vi "create table discretes.vi"(10 "DI table":string[](array[string]), 11 "table name":string="XB") -> (3 "create table parameters":string)   [LabVIEW 2019, in "PostgreSQL.lvlib"]
uses:
  PostgreSQL.lvlib
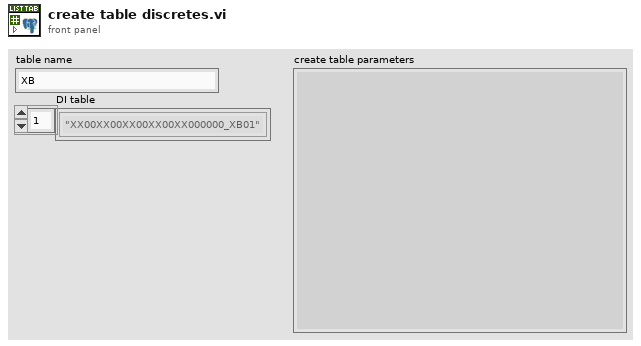
[diagram p1: front panel]
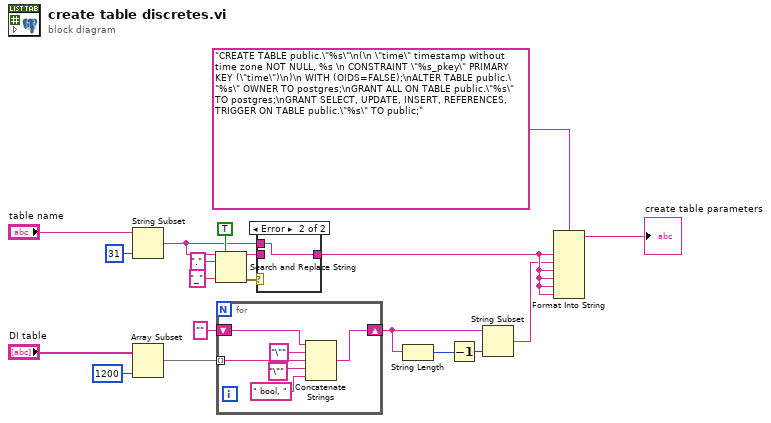
[diagram p0: block diagram]
diagram:
  n1 = String Subset(string="table name", length (rest)=31 ("offset (0)")) -> (substring=w14:string)  [unwired: 1 in]
  n2 = Array Subset(array="DI table", length=1200) -> (w2:string[])  [unwired: 1 in]
  n3 = Search and Replace String(replace all?=TRUE ("replace all? (F)"), input string=w14, search string=".", replace string="_" ("replace string (\"\")")) -> (result string=w16:string, error out=w17:errorcluster)  [unwired: 4 in, 2 out]
  n4 = for {
    tunnel: w2 -> [w23] mode=indexing
    shift-right: [w20] -> w4
    shift-left: "" ("result string") -> [w21]
    n5 = Concatenate Strings(w21, "\"" ("string"), w23, "\"" ("string"), " bool, ") -> (w20:string)
  }
  n6 = case shown="Error" w17 {
    tunnel: w16 -> [w26 _]
    tunnel: [w26 w27] -> w9
    tunnel: w14 -> [_ w27]
    frame No Error {
    }
    frame Error {
    }
  }
  n7 = String Length(string=w4) -> (length=w3:i32)
  n8 = Decrement(x=w3) -> (x-1=w6:i32)
  n9 = String Subset(string=w4, length (rest)=w6) -> (substring=w1:string)  [unwired: 1 in]
  n10 = Format Into String(format string="CREATE TABLE public.\"%s\"\n(\n \"time\" timestamp without time zone NOT NULL, %s \n CONSTRAINT \"%s_pkey\" PRIMARY KEY (\"time\")\n)\n WITH (OIDS=FALSE);\nALTER TABLE public.\"%s\" OWNER TO postgres;\nGRANT ALL ON TABLE public.\"%s\" TO postgres;\nGRANT SELECT, UPDATE, INSERT, REFERENCES, TRIGGER ON TABLE public.\"%s\" TO public;", w9, w1, w9, w9, w9, w9) -> (resulting string=→"create table parameters":string)  [unwired: 2 in, 1 out]
